vi "Pulse Timer（Tool)vi.vi"(8 "error in":errorcluster, 9 "preset time (ms)":u32=1000, 11 "input":bool) -> (0 "error out":errorcluster, 1 "elapsed time (ms)":u32, 3 "output":bool)   [LabVIEW 2012, in "毫秒定时器.lvlib"]
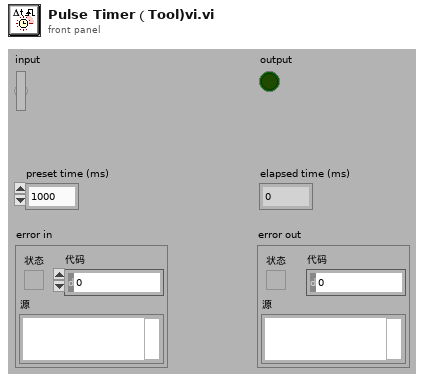
[diagram p1: front panel]
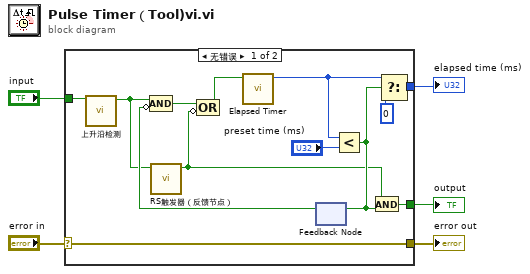
[diagram p0: block diagram]
diagram:
  n1 = case shown="无错误" "error in" {
    selector: "error in" -> [w18 w19]
    tunnel: [w18 w19] -> w4
    tunnel: "input" -> [w7 _]
    tunnel: [w12 _] -> w2
    tunnel: [w10 _] -> w1
    frame No Error {
      n2 = call "上升沿检测.vi"("input"=w7) -> ("output"=w6:bool)  [unwired: 9 in, 1 out]
      n3 = call "RS触发器（反馈节点）.vi"("S"=w6) -> ("Q"=w11:bool)  [unwired: 10 in]
      n4 = feedback #1() -> (w14:bool)  [unwired: 1 in]
      n5 = Compound Arithmetic op=AND(w6, invert w14) -> (w13:bool)
      n6 = Compound Arithmetic op=OR(w13, invert w11) -> (w9:bool)
      n7 = call "Elapsed Timer.vi"("reset"=w9) -> ("elapsed time"=w8:u32)  [unwired: 8 in, 2 out]
      n8 = Less?(x=w8, y="preset time (ms)") -> (x < y?=w16:bool)
      n9 = feedback-in #1(w16) -> ()
      n10 = And(x=w11, y=w16) -> (x .and. y?=w10:bool)
      n11 = Select(t=w8, s=w16, f=u32 0) -> (s? t:f=w12:u32)
    }
    frame Error {
    }
  }
  "error out" <- w4
  "elapsed time (ms)" <- w2
  "output" <- w1
